vi "Rcalc.vi"() -> ()   [LabVIEW 2019]
uses:
  <userlib>/caLab/Private/Get_PV-1D.vi
  <userlib>/caLab/Private/Put_DBL-1D_PV-1D.vi
panel:
  in  "Boolean":bool
  out "x/y":dbl
  in  "I":dbl
  in  "V":dbl
  out "APX:Theater":dbl
  in  "APX:PS2_Rzero":dbl
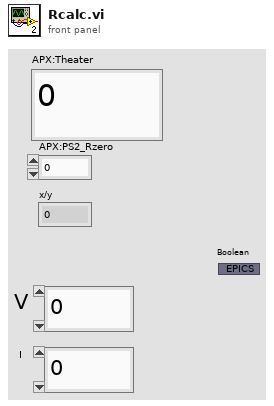
[diagram p1: front panel]
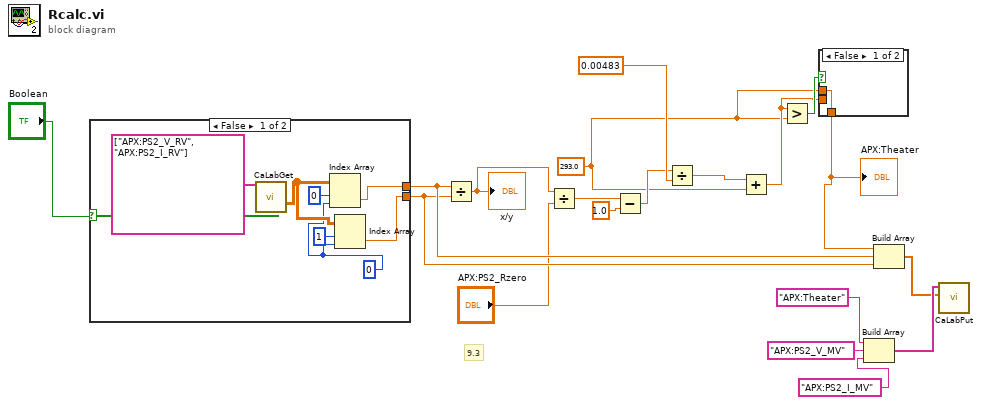
[diagram p0: block diagram]
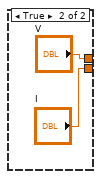
[diagram p3: hidden frame]
diagram:
  w1 = 293.0 ("y")
  # "9.3"
  n1 = case shown="False" "Boolean" {
    tunnel: [w21 "V"] -> w9
    tunnel: [w22 "I"] -> w8
    frame False {
      w20 = 0 ("index (col)")
      n2 = call-poly <userlib>:"CaLabGet.vi"("PV Names"=string[] ["APX:PS2_V_RV", "APX:PS2_I_RV"]) -> ("Value Array (number)"=w26:dbl[][])  [unwired: 8 in, 6 out]
      n3 = Index Array(array=w26, index (row)=0 ("disabled index (row)"), index (col)=w20) -> (element=w21:dbl)
      n4 = Index Array(array=w26, index (row)=1, index (col)=w20) -> (element=w22:dbl)
    }
    frame True {
    }
  }
  n5 = Divide(x=w9, y=w8) -> (x/y=w14:dbl)
  "x/y" <- w14
  n6 = Divide(x=w14, y="APX:PS2_Rzero") -> (x/y=w19:dbl)
  n7 = Subtract(x=w19, y=1.0) -> (x-y=w15:dbl)
  n8 = Divide(x=w15, y=0.00483 ("APX:PS2_Ct")) -> (x/y=w17:dbl)
  n9 = Add(x=w17, y=w1) -> (x+y=w2:dbl)
  n10 = Greater?(x=w2, y=w1) -> (0:w4:bool)
  n11 = case shown="False" w4 {
    tunnel: w2 -> [_ w30]
    tunnel: [w29 w30] -> w3
    tunnel: w1 -> [w29 _]
    frame False {
    }
    frame True {
    }
  }
  "APX:Theater" <- w3
  n12 = Build Array("APX:Theater" ("PV Name"), "APX:PS2_V_MV" ("element"), "APX:PS2_I_MV" ("element")) -> (w10:string[])
  n13 = Build Array(w3, w9, w8) -> (w7:dbl[])
  n14 = call-poly <userlib>:"CaLabPut.vi"("Values"=w7, "PV Names"=w10) -> ()  [unwired: 6 in, 4 out]
